vi "Lorentzian complex bg test.vi"(3 "output control":T1, 4 "data":variant, 5 "X":dbl[](array[numeric]), 6 "a":dbl[](array[numeric])) -> (0 "error out":errorcluster, 1 "f'(X,a)":dbl[][](array[numeric]), 2 "f(X,a)":dbl[](array[numeric]))   [LabVIEW 2016]
doc: "Sum of three Gaussians, plus DC offset."
uses:
  <vilib>/gmath/NumericalOptimization/LM_output select.ctl
  <vilib>/gmath/NI_Gmath.lvlib
panel:
  out "Waveform Graph":dbl[](graph)
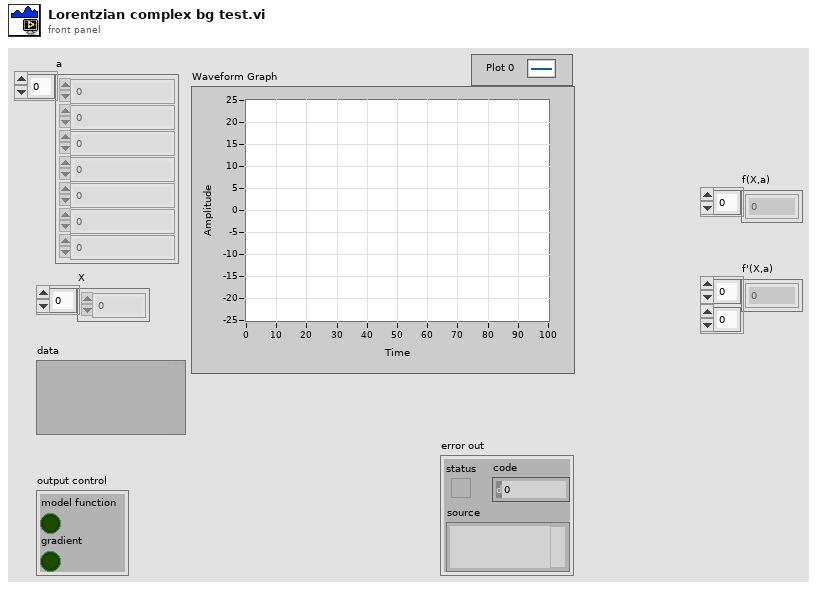
[diagram p1: front panel]
types:
  T1 = typedef "NI_Gmath.lvlib/LM_output select.ctl" = cluster{"model function":bool, "gradient":bool}
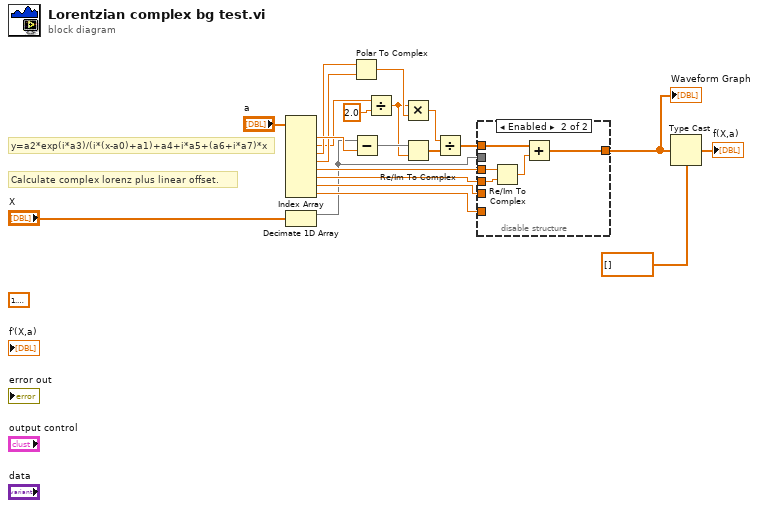
[diagram p0: block diagram]
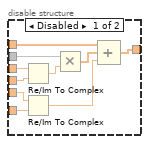
[diagram p2: hidden frame]
diagram:
  (unwired) 1.5707963267948966
  # "y=a2*exp(i*a3)/(i*(x-a0)+a1)+a4+i*a5+(a6+i*a7)*x"
  # "Calculate complex lorenz plus linear offset."
  n1 = Index Array(array="a") -> (element #1=w20:dbl, element #2=w2:dbl, element #3=w17:dbl, element #4=w16:dbl, element #5=w14:dbl, element #6=w13:dbl, element #7=w11:dbl, element #8=w10:dbl)  [unwired: 8 in]
  n2 = Decimate 1D Array("X") -> (w8:dbl[])  [unwired: 1 out]
  n3 = Polar To Complex(1:w16, 2:w17) -> (0:w19:cdb)
  n4 = Subtract(x=w8, y=w20) -> (x-y=w5:dbl[])
  n5 = Divide(x=w2, y=2.0) -> (x/y=w1:dbl)
  n6 = Multiply(x=w1, y=w19) -> (x*y=w4:cdb)
  n7 = Re/Im To Complex(1:w1, 2:w5) -> (0:w18:cdb[])
  n8 = Divide(x=w4, y=w18) -> (x/y=w9:cdb[])
  n9 = disable-structure shown="Enabled" {
    disable-tunnel: w14 -> [w31 w36]
    disable-tunnel: w13 -> [w30 w35]
    disable-tunnel: w11 -> [w27 _]
    disable-tunnel: w10 -> [w26 _]
    disable-tunnel: w9 -> [w24 w34]
    disable-tunnel: [w23 w33] -> w6
    disable-tunnel: w8 -> [w22 _]
    frame Disabled {
      n10 = Re/Im To Complex(1:w30, 2:w31) -> (0:w29:cdb)
      n11 = Re/Im To Complex(1:w26, 2:w27) -> (0:w25:cdb)
      n12 = Multiply(x=w22, y=w29) -> (x*y=w28:cdb[])
      n13 = Compound Arithmetic op=ADD(w24, w28, w25) -> (w23:cdb[])
    }
    frame Enabled {
      n14 = Re/Im To Complex(1:w35, 2:w36) -> (0:w32:cdb)
      n15 = Add(x=w34, y=w32) -> (x+y=w33:cdb[])
    }
  }
  "Waveform Graph" <- w6
  n16 = Type Cast(type=dbl[] [], x=w6) -> (*(type *) &x=→"f(X,a)":dbl[])
